vi "规范小时时间戳.vi"(11 "字符串":string) -> (3 "result string":string)   [LabVIEW 2016, in "数据传输系统-04.lvlib"]
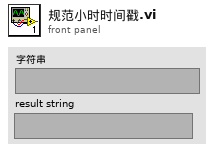
[diagram p1: front panel]
types:
  T1 = typedef "LVDateTimeRec.ctl" = cluster{"秒数的小数部分":dbl, "秒":i32, "分":i32, "时":i32, "日":i32, "月":i32, "年":i32, "天数（周）":i32, "天数（年）":i32, "DST":i32}
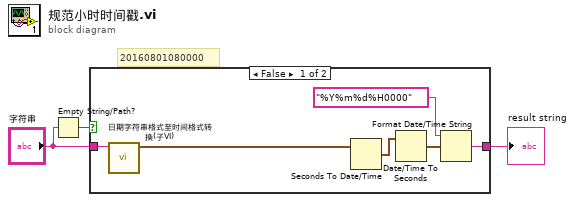
[diagram p0: block diagram]
diagram:
  # "20160801080000"
  n1 = Empty String/Path?(string/path="字符串") -> (empty?=w1:bool)
  n2 = case shown="False" w1 {
    tunnel: "字符串" -> [w6 w10]
    tunnel: [w5 w10] -> w3
    frame False {
      n3 = call "日期字符串格式至时间格式转换(子VI).vi"("data[0]"=w6) -> ("time stamp"=w7:timestamp)  [unwired: 10 in]
      n4 = Seconds To Date/Time(time stamp (now)=w7) -> (date time rec=w4:T1)  [unwired: 1 in]
      n5 = Date/Time To Seconds(2:w4) -> (0:w8:timestamp)  [unwired: 1 in]
      n6 = Format Date/Time String(time format string (%c)="%Y%m%d%H0000" ("时间格式字符串(%c)"), seconds (now)=w8) -> (date/time string=w5:string)  [unwired: 1 in]
    }
    frame True {
    }
  }
  "result string" <- w3
